vi "SPARK Configure Power.vi"   [LabVIEW 2023]
doc: "Configure power settings of the SPARK."
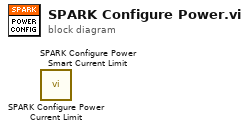
[diagram p0: block diagram]
diagram:
  n1 = call "SPARK Configure Power Current Limit.vi"() -> ()  [unwired: 10 in, 2 out]
  n2 = call "SPARK Configure Power Smart Current Limit.vi"() -> ()  [unwired: 10 in, 2 out]
